vi "~Listbox for Atten and Phase Shift.vi"() -> ()   [LabVIEW 2017]
panel:
  in  "Phase Shift":i32[](listbox)
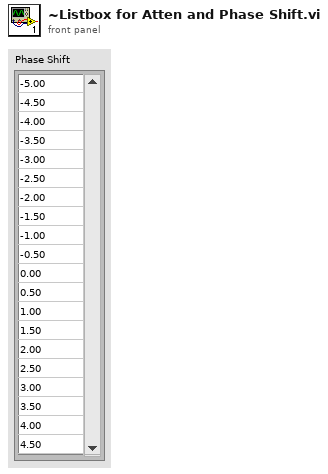
[diagram p1: front panel]
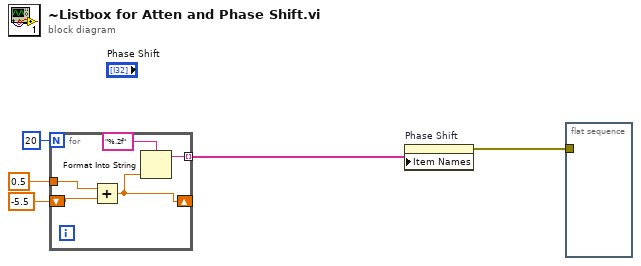
[diagram p0: block diagram]
diagram:
  n1 = for {
    N: 20 -> [_]
    shift-right: [w8] -> _
    shift-left: -5.5 -> [w10]
    tunnel: 0.5 -> [w9]
    tunnel: [w6] -> w2 mode=indexing
    n2 = Add(x=w9, y=w10) -> (x+y=w8:dbl)
    n3 = Format Into String(format string="%.2f", w8) -> (resulting string=w6:string)  [unwired: 2 in, 1 out]
  }
  n4 = property on="Phase Shift" class="LstBox (strict)"("Item Names"=w2) -> (error out=w1:errorcluster)  [unwired: 2 in, 1 out]
  n5 = flat-sequence {
    tunnel: w1 -> [_]
    frame #0 {
    }
  }
